vi "Arduino UART loop.vi"() -> ()   [LabVIEW 2017]
uses:
  <vilib>/myRIO/Instrument Drivers/Onboard IO/UART/typedef/VISA Configuration.ctl
  <vilib>/myRIO/Instrument Drivers/Onboard IO/UART/UART.lvlib
panel:
  out "error?":bool
  in  "stop":bool
  out "read buffer":string
  in  "Read mode":enum16{"Read all", "Get latest value"}(ring)=enum."Get latest value"
  in  "VISA resource name in":refnum<visa-resource-name>="ASRL1::INSTR"
  out "timeout (10sec)":u32
  in  "input cluster":T1={"baud rate (9600)"=115200, "data bits (8)"=8, "parity (0:none)"=enum."None", "stop bits (10: 1 bit)"=10, "flow control (0:none)"=0, "termination char\n(0xA = '\\n' = LF) "=10, "Enable Termination\nChar (T)"=TRUE, "timeout (10sec)"=1000} {"termination char\n(0xA = '\\n' = LF)" format="%.0x"; "flow control (0:none)" items=["None", "XON/XOFF", "RTS/CTS", "XON/XOFF & RTS/CTS", "DTR/DSR", "XON/XOFF & DTR/DSR"]; "stop bits (10: 1 bit)" items=["1.0"=10, "1.5"=15, "2.0"=20]; "data bits (8)" min=5 max=8 step=1}
  out "error out":errorcluster
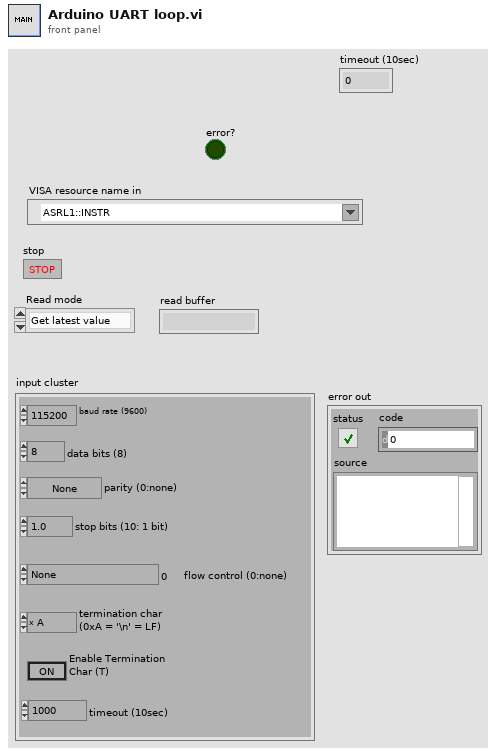
[diagram p1: front panel]
types:
  T1 = typedef "UART.lvlib/VISA Configuration.ctl" = cluster{"baud rate (9600)":u32, "data bits (8)":u16, "parity (0:none)":enum16{"None", "Odd", "Even", "Mark", "Space"}, "stop bits (10: 1 bit)":u16, "flow control (0:none)":u16, "termination char\n(0xA = '\\n' = LF) ":u8, "Enable Termination\nChar (T)":bool, "timeout (10sec)":u32}
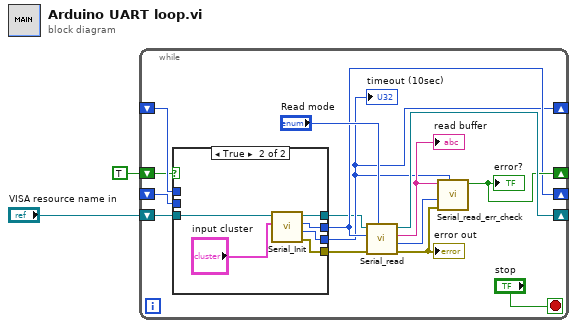
[diagram p0: block diagram]
diagram:
  n1 = while {
    shift-right: [w16] -> _
    shift-left: "VISA resource name in" -> [w5]
    shift-right: [w12] -> _
    shift-left: TRUE ("error?") -> [w4]
    shift-right: [w10] -> _
    shift-left: _ -> [w9]
    shift-right: [w8] -> _
    shift-left: _ -> [w7]
    stop <- "stop" stop-if-true
    n2 = case shown="True" w4 {
      tunnel: [_ w25] -> w11
      tunnel: [w19 w24] -> w8
      tunnel: [w20 w23] -> w10
      tunnel: w9 -> [w20 _]
      tunnel: w7 -> [w19 _]
      tunnel: [w18 w22] -> w6
      tunnel: w5 -> [w18 w21]
      frame False {
      }
      frame True {
        n3 = call "Serial_Init.vi"("input cluster"="input cluster", "VISA Refnum in"=w21) -> ("error out"=w25:errorcluster, "timeout (10sec)"=w24:u32, "Bytes at Port"=w23:u32, "VISA Refnum out"=w22:refnum<visa-resource-name>)  [unwired: 6 in]
      }
    }
    "timeout (10sec)" <- w8
    n4 = call "Serial_read.vi"("Read mode"="Read mode", "error in (no error)"=w11, "Bytes at Port"=w10, "VISA Refnum in"=w6) -> ("error out"=w14:errorcluster, "dt"=w13:u32, "read buffer"=w15:string, "VISA resource name out"=w16:refnum<visa-resource-name>)  [unwired: 4 in]
    "error out" <- w14
    "read buffer" <- w15
    n5 = call "Serial_read_err_check.vi"("timeout"=w8, "error in (no error)"=w14, "dt"=w13, "read buffer"=w15) -> ("error?"=w12:bool)  [unwired: 7 in]
    "error?" <- w12
  }
